vi "Simulador OPC.vi"(0 "String vindo do labview":string, 1 "String vindo do CLP":string) -> (3 "String para labview 12":string, 4 "String para labview 11":string, 5 "String para labview 10":string, 7 "String para labview 9":string, 9 "String para labview 8":string, 11 "String para labview 7":string, 13 "String para labview 6":string, 14 "String para CLP":string, 15 "String para labview 1":string, 16 "String para labview 2":string, 17 "String para labview 3":string, 18 "String para labview 4":string, 19 "String para labview 5":string)   [LabVIEW 2019]
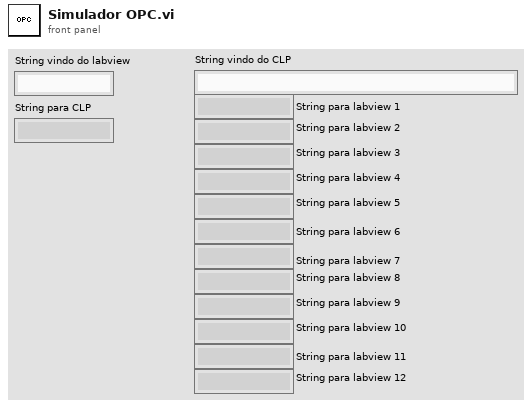
[diagram p1: front panel]
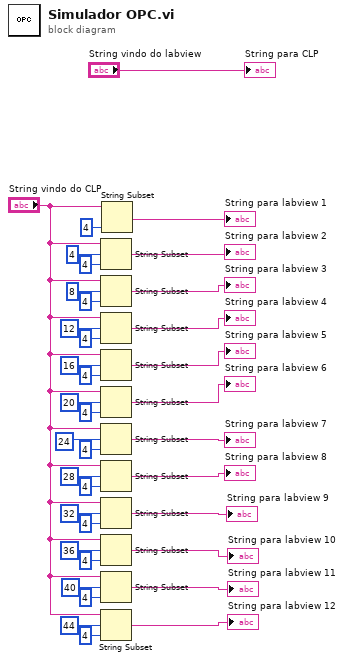
[diagram p0: block diagram]
diagram:
  n1 = String Subset(string="String vindo do CLP", offset (0)=4, length (rest)=4 ("length (rest)")) -> (substring=→"String para labview 2":string)
  n2 = String Subset(string="String vindo do CLP", offset (0)=8, length (rest)=4 ("length (rest)")) -> (substring=→"String para labview 3":string)
  n3 = String Subset(string="String vindo do CLP", offset (0)=12, length (rest)=4 ("length (rest)")) -> (substring=→"String para labview 4":string)
  n4 = String Subset(string="String vindo do CLP", offset (0)=16, length (rest)=4 ("length (rest)")) -> (substring=→"String para labview 5":string)
  n5 = String Subset(string="String vindo do CLP", offset (0)=20, length (rest)=4 ("length (rest)")) -> (substring=→"String para labview 6":string)
  n6 = String Subset(string="String vindo do CLP", offset (0)=24 ("length (rest)"), length (rest)=4 ("length (rest)")) -> (substring=→"String para labview 7":string)
  n7 = String Subset(string="String vindo do CLP", offset (0)=28, length (rest)=4 ("length (rest)")) -> (substring=→"String para labview 8":string)
  n8 = String Subset(string="String vindo do CLP", offset (0)=32, length (rest)=4 ("length (rest)")) -> (substring=→"String para labview 9":string)
  n9 = String Subset(string="String vindo do CLP", offset (0)=36, length (rest)=4 ("length (rest)")) -> (substring=→"String para labview 10":string)
  n10 = String Subset(string="String vindo do CLP", offset (0)=40, length (rest)=4 ("length (rest)")) -> (substring=→"String para labview 11":string)
  n11 = String Subset(string="String vindo do CLP", offset (0)=44, length (rest)=4 ("length (rest)")) -> (substring=→"String para labview 12":string)
  n12 = String Subset(string="String vindo do CLP", length (rest)=4 ("length (rest)")) -> (substring=→"String para labview 1":string)  [unwired: 1 in]
  "String para CLP" <- "String vindo do labview"
